vi "UpdateOneStep.vi"(8 "error in (no error)":errorcluster, 11 "OneStep?":bool) -> (0 "error out":errorcluster)   [LabVIEW 2016, in "SeqProcessor.lvlib"]
uses:
  SeqProcessor.lvlib
  <vilib>/addons/PointValueMap/subVIs/Point_Write_variant.vi
  <vilib>/addons/PointValueMap/PointValueMap.lvlib
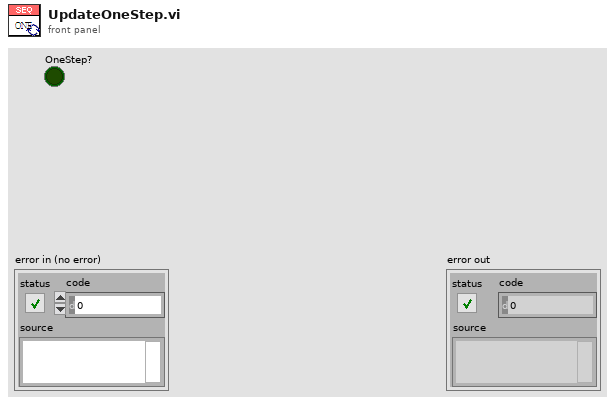
[diagram p1: front panel]
types:
  T1 = typedef "PointValueMap.lvlib/PointMap.ctl" = refnum<data-value>
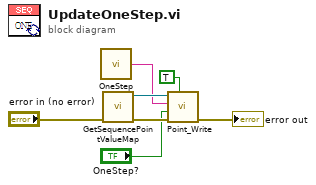
[diagram p0: block diagram]
diagram:
  n1 = call "OneStep.vi"() -> ("OneStep"=w3:string)  [unwired: 5 in]
  n2 = call "GetSequencePointValueMap.vi"("error in (no error)"="error in (no error)") -> ("error out"=w5:errorcluster, "SeqMap"=w4:T1)  [unwired: 9 in]
  n3 = call-poly <vilib>:"Point_Write.vi"("Auto Create?"=TRUE, "Error In"=w5, "Value"="OneStep?", "Tag"=w3, "Map"=w4) -> ("Error Out"=→"error out":errorcluster)  [unwired: 5 in, 1 out]
